vi "Lab1.0.vi"() -> ()   [LabVIEW 2024]
panel:
  in  "Force Speed":string(combo)="XAg"
  out "Time(ms)":dbl=1.489 format="%<%H:%M:%S%3u>t"
  in  "Secondary Parameter":string(combo)=":CALC2:FORM Q"
  in  "Primary Parameter":string(combo)=":CALC1:FORM R"
  in  "LCR Speed":string(combo)=":APER MED"
  in  "STOP Mesurement":bool caption="stop"
  out "Status":bool=TRUE
  in  "Stop Main Loop":bool
  in  "Sample Rate":dbl=10.0 min=0.0001 max=500.0
  out "Position":dbl=-25869.0
  out "Force":dbl
  out "Secondary Parameter":dbl=165.48 format="%#_6p"
  out "Primary Parameter":dbl=23864000000.0 format="%#_6p"
  in  "Mesurement":bool caption="stop"
  out "Origin Data  From Force Measurement":string
  in  "Force Measurement":refnum<visa-resource-name>
  out "Origin Data From LCR Meter":string="+0,+2.38640E+10,+1.65480E+02\n"
  in  "LCR Meter":refnum<visa-resource-name>
  # "Hz"
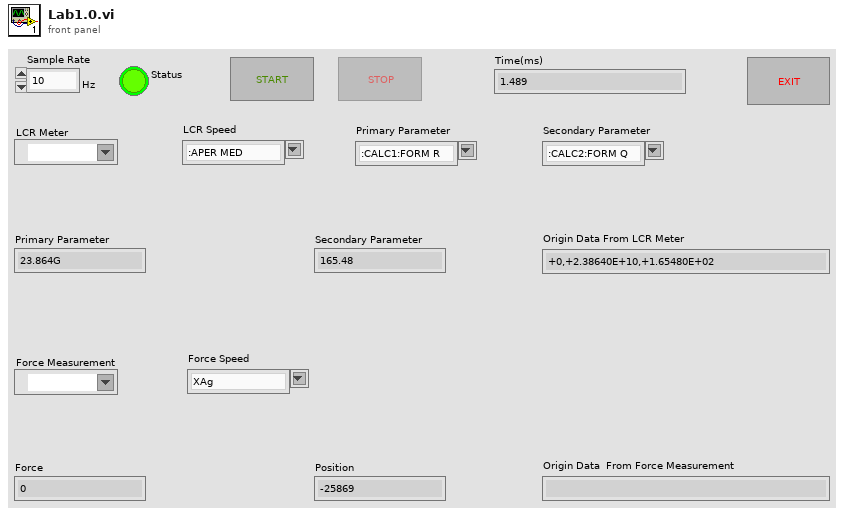
[diagram p1: front panel]
types:
  T1 = enum16{"open", "replace", "create", "open or create", "replace or create", "replace or create with confirmation"}
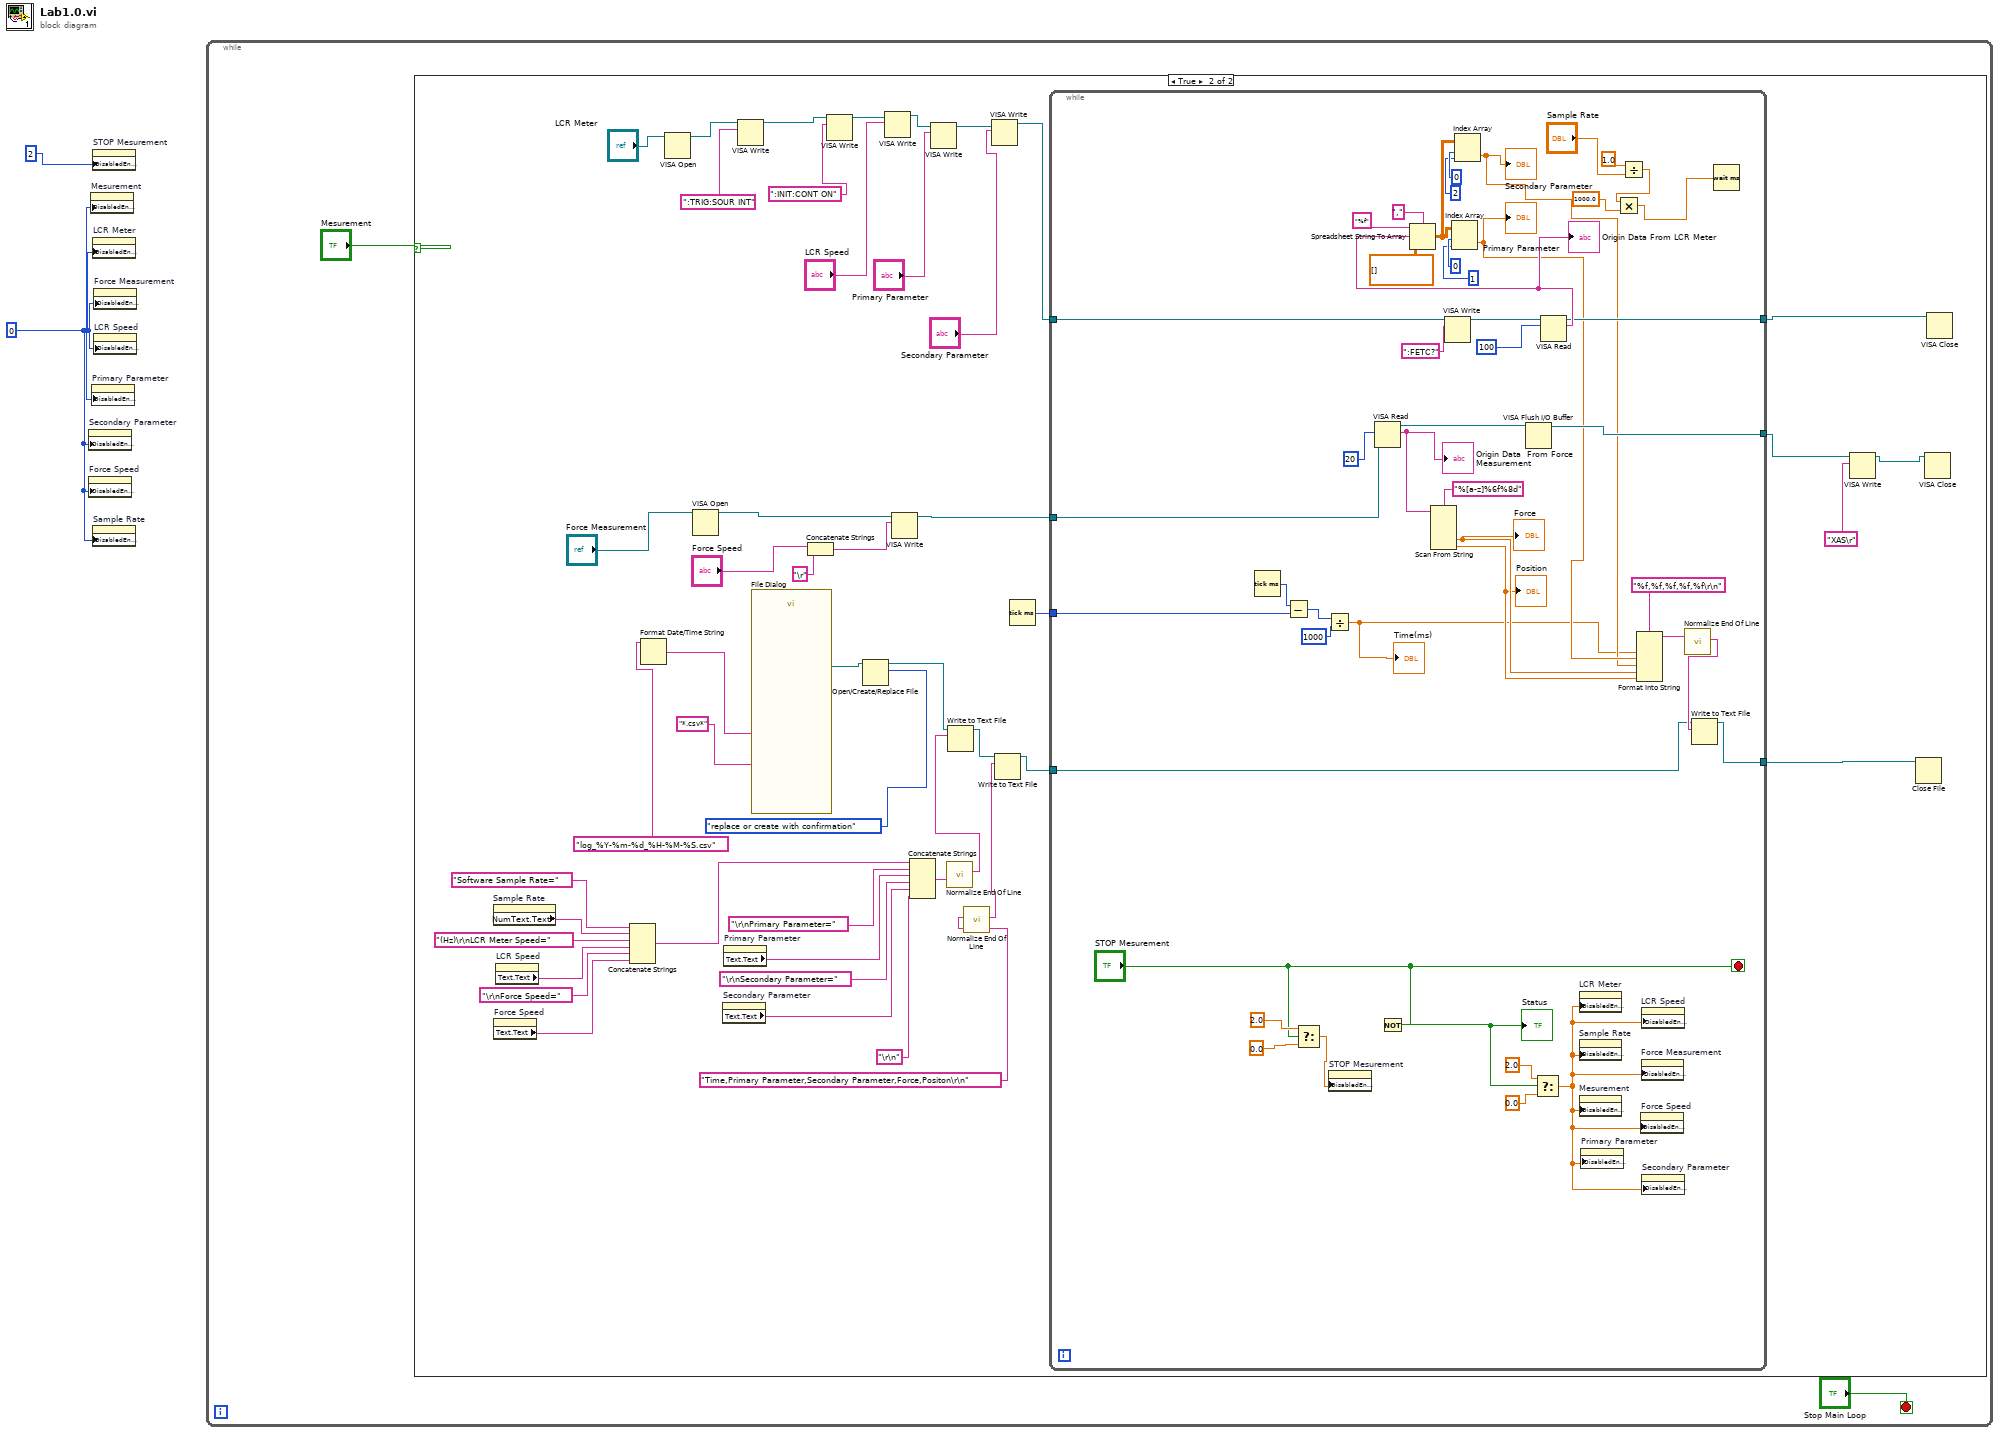
[diagram p0: block diagram]
diagram:
  w1 = 0
  n1 = property on="Secondary Parameter" class="CmbBox"("DisabledEnum"=w1) -> ()  [unwired: 2 in, 2 out]
  n2 = property on="Force Speed" class="CmbBox"("DisabledEnum"=w1) -> ()  [unwired: 2 in, 2 out]
  n3 = property on="Mesurement" class="Bool"("DisabledEnum"=w1) -> ()  [unwired: 2 in, 2 out]
  n4 = property on="Primary Parameter" class="CmbBox"("DisabledEnum"=w1) -> ()  [unwired: 2 in, 2 out]
  n5 = property on="STOP Mesurement" class="Bool"("DisabledEnum"=2) -> ()  [unwired: 2 in, 2 out]
  n6 = property on="LCR Meter" class="VISAName"("DisabledEnum"=w1) -> ()  [unwired: 2 in, 2 out]
  n7 = property on="Sample Rate" class="DigNum (strict)"("DisabledEnum"=w1) -> ()  [unwired: 2 in, 2 out]
  n8 = property on="Force Measurement" class="VISAName"("DisabledEnum"=w1) -> ()  [unwired: 2 in, 2 out]
  n9 = property on="LCR Speed" class="CmbBox"("DisabledEnum"=w1) -> ()  [unwired: 2 in, 2 out]
  n10 = while {
    stop <- "Stop Main Loop" stop-if-true
    n11 = case shown="True" "Mesurement" {
      frame False {
      }
      frame True {
        n12 = property on="Sample Rate" class="DigNum (strict)"() -> ("NumText.Text"=w10:string)  [unwired: 2 in, 2 out]
        n13 = property on="Force Speed" class="CmbBox"() -> ("Text.Text"=w6:string)  [unwired: 2 in, 2 out]
        n14 = property on="LCR Speed" class="CmbBox"() -> ("Text.Text"=w8:string)  [unwired: 2 in, 2 out]
        n15 = Concatenate Strings("Software Sample Rate=" ("text"), w10, "(Hz)\r\nLCR Meter Speed=" ("text"), w8, "\r\nForce Speed=" ("text"), w6) -> (w5:string)
        n16 = Format Date/Time String(time format string (%c)="log_%Y-%m-%d_%H-%M-%S.csv") -> (date/time string=w38:string)  [unwired: 2 in]
        n17 = VISA Open(VISA resource name="LCR Meter") -> (VISA resource name=w51:refnum<visa-resource-name>)  [unwired: 4 in, 1 out]
        n18 = VISA Open(VISA resource name="Force Measurement") -> (VISA resource name=w44:refnum<visa-resource-name>)  [unwired: 4 in, 1 out]
        n19 = property on="Secondary Parameter" class="CmbBox"() -> ("Text.Text"=w22:string)  [unwired: 2 in, 2 out]
        n20 = property on="Primary Parameter" class="CmbBox"() -> ("Text.Text"=w20:string)  [unwired: 2 in, 2 out]
        n21 = VISA Write(VISA resource name=w51, write buffer=":TRIG:SOUR INT") -> (VISA resource name out=w49:refnum<visa-resource-name>)  [unwired: 1 in, 2 out]
        n22 = call "File Dialog"("default name"=w38, "pattern (all files)"="*.csv*") -> ("selected path"=w37:path)  [unwired: 10 in, 3 out]
        n23 = Concatenate Strings("Force Speed", "\r" ("string")) -> (w14:string)
        n24 = VISA Write(VISA resource name=w49, write buffer=":INIT:CONT ON") -> (VISA resource name out=w47:refnum<visa-resource-name>)  [unwired: 1 in, 2 out]
        n25 = Open/Create/Replace File(file path (use dialog)=w37, operation (0:open)=T1."replace or create with confirmation") -> (refnum out=w25:refnum<file>)  [unwired: 4 in, 2 out]
        n26 = VISA Write(VISA resource name=w47, write buffer="LCR Speed") -> (VISA resource name out=w46:refnum<visa-resource-name>)  [unwired: 1 in, 2 out]
        n27 = VISA Write(VISA resource name=w44, write buffer=w14) -> (VISA resource name out=w42:refnum<visa-resource-name>)  [unwired: 1 in, 2 out]
        n28 = Concatenate Strings(w5, "\r\nPrimary Parameter=" ("text"), w20, "\r\nSecondary Parameter=" ("text"), w22, "\r\n" ("text")) -> (w18:string)
        n29 = VISA Write(VISA resource name=w46, write buffer="Primary Parameter") -> (VISA resource name out=w45:refnum<visa-resource-name>)  [unwired: 1 in, 2 out]
        n30 = call <vilib>:"Normalize End Of Line.vi"("string in"=w18) -> ("string out"=w17:string)  [unwired: 7 in]
        n31 = Write to Text File(file (use dialog)=w25, text=w17) -> (refnum out=w24:refnum<file>)  [unwired: 2 in, 2 out]
        n32 = call <vilib>:"Normalize End Of Line.vi"("string in"="Time,Primary Parameter,Secondary Parameter,Force,Positon\r\n" ("text")) -> ("string out"=w29:string)  [unwired: 7 in]
        n33 = VISA Write(VISA resource name=w45, write buffer="Secondary Parameter") -> (VISA resource name out=w41:refnum<visa-resource-name>)  [unwired: 1 in, 2 out]
        n34 = Write to Text File(file (use dialog)=w24, text=w29) -> (refnum out=w13:refnum<file>)  [unwired: 2 in, 2 out]
        n35 = Tick Count (ms)() -> (millisecond timer value=w12:u32)
        n36 = while {
          tunnel: [w94] -> w39
          tunnel: w42 -> [w96]
          tunnel: w41 -> [w76]
          tunnel: [w75] -> w33
          tunnel: [w74] -> w31
          tunnel: w13 -> [w54]
          tunnel: w12 -> [w53]
          stop <- "STOP Mesurement" stop-if-true
          n37 = Tick Count (ms)() -> (millisecond timer value=w63:u32)
          n38 = Subtract(x=w63, y=w53) -> (x-y=w58:u32)
          n39 = Select(t=2.0, s="STOP Mesurement", f=0.0) -> (s? t:f=w59:dbl)
          n40 = Divide(x=w58, y=u32 1000) -> (x/y=w56:dbl)
          "Time(ms)" <- w56
          n41 = property on="STOP Mesurement" class="Bool"("DisabledEnum"=w59) -> ()  [unwired: 2 in, 2 out]
          n42 = VISA Read(VISA resource name=w96, byte count=u32 20) -> (VISA resource name out=w95:refnum<visa-resource-name>, read buffer=w83:string)  [unwired: 1 in, 2 out]
          "Origin Data  From Force Measurement" <- w83
          n43 = Not(x="STOP Mesurement") -> (.not. x?=w64:bool)
          "Status" <- w64
          n44 = Scan From String(format string="%[a-z]%6f%8d", input string=w83) -> (output 2=w71:dbl, output 3=w70:dbl)  [unwired: 6 in, 3 out]
          "Force" <- w71
          "Position" <- w70
          n45 = VISA Write(VISA resource name=w76, write buffer=":FETC?") -> (VISA resource name out=w99:refnum<visa-resource-name>)  [unwired: 1 in, 2 out]
          n46 = VISA Flush I/O Buffer(VISA resource name=w95) -> (VISA resource name out=w94:refnum<visa-resource-name>)  [unwired: 2 in, 1 out]
          n47 = Select(t=2.0, s=w64, f=0.0) -> (s? t:f=w55:dbl)
          n48 = VISA Read(VISA resource name=w99, byte count=u32 100) -> (VISA resource name out=w75:refnum<visa-resource-name>, read buffer=w92:string)  [unwired: 1 in, 2 out]
          "Origin Data From LCR Meter" <- w92
          n49 = Spreadsheet String To Array(delimiter (Tab)=",", format string="%f", spreadsheet string=w92, array type (2D Dbl)=dbl[][] []) -> (array=w86:dbl[][])
          n50 = Index Array(array=w86, index (row)=0 ("index"), index (col)=1) -> (element=w73:dbl)
          "Primary Parameter" <- w73
          n51 = Index Array(array=w86, index (row)=0, index (col)=2) -> (element=w72:dbl)
          "Secondary Parameter" <- w72
          n52 = property on="LCR Meter" class="VISAName"("DisabledEnum"=w55) -> ()  [unwired: 2 in, 2 out]
          n53 = property on="Sample Rate" class="DigNum (strict)"("DisabledEnum"=w55) -> ()  [unwired: 2 in, 2 out]
          n54 = property on="Mesurement" class="Bool"("DisabledEnum"=w55) -> ()  [unwired: 2 in, 2 out]
          n55 = property on="Primary Parameter" class="CmbBox"("DisabledEnum"=w55) -> ()  [unwired: 2 in, 2 out]
          n56 = Divide(x=1.0, y="Sample Rate") -> (x/y=w78:dbl)
          n57 = Multiply(x=w78, y=1000.0) -> (x*y=w79:dbl)
          n58 = Format Into String(format string="%f,%f,%f,%f,%f\r\n", w56, w73, w72, w71, w70) -> (resulting string=w68:string)  [unwired: 2 in, 1 out]
          n59 = property on="Force Speed" class="CmbBox"("DisabledEnum"=w55) -> ()  [unwired: 2 in, 2 out]
          n60 = property on="Force Measurement" class="VISAName"("DisabledEnum"=w55) -> ()  [unwired: 2 in, 2 out]
          n61 = property on="LCR Speed" class="CmbBox"("DisabledEnum"=w55) -> ()  [unwired: 2 in, 2 out]
          n62 = property on="Secondary Parameter" class="CmbBox"("DisabledEnum"=w55) -> ()  [unwired: 2 in, 2 out]
          n63 = call <vilib>:"Normalize End Of Line.vi"("string in"=w68) -> ("string out"=w67:string)  [unwired: 7 in]
          n64 = Write to Text File(file (use dialog)=w54, text=w67) -> (refnum out=w74:refnum<file>)  [unwired: 2 in, 2 out]
          n65 = Wait (ms)(milliseconds to wait=w79) -> ()  [unwired: 1 out]
        }
        n66 = VISA Write(VISA resource name=w39, write buffer="XAS\r") -> (VISA resource name out=w32:refnum<visa-resource-name>)  [unwired: 1 in, 2 out]
        n67 = Close File(refnum=w31) -> ()  [unwired: 1 in, 2 out]
        n68 = VISA Close(VISA resource name=w32) -> ()  [unwired: 1 in, 1 out]
        n69 = VISA Close(VISA resource name=w33) -> ()  [unwired: 1 in, 1 out]
      }
    }
  }
